vi "MFP3D Acquired Data.vi"() -> ()   [LabVIEW 2016]
uses:
  <userlib>/LevyLab/Relay Box/Type_defs/Resistor--enum.ctl
  <vilib>/DAQmx/read.llb/DAQmx Read (Analog 1D DBL NChan 1Samp).vi
  subVIs/Driver Variables_MFP3D.vi
  <vilib>/DAQmx/create/channels.llb/DAQmx Create Channel (AI-Voltage-Basic).vi
  <vilib>/DAQmx/configure/timing.llb/DAQmx Timing (Sample Clock).vi
  <vilib>/DAQmx/miscellaneous.llb/DAQmx Fill In Error Info.vi
  <vilib>/Platform/TimedLoop/XDataNode/XDataNode.xnode
  <vilib>/Platform/TimedLoop/XDataNode/timing_clust.ctl
  <vilib>/Platform/TimedLoop/XDataNode/nitl_modes.ctl
  <vilib>/Platform/TimedLoop/XDataNode/wakeup.ctl
  <vilib>/Platform/TimedLoop/XDataNode/XDNodeRunTimeDep.lvlib
panel:
  in  "Reset Graphs":bool
  in  "Data Queue":refnum<queue>
  in  "Skip Back Button":bool
  in  "FF Speed":dbl=2.0
  in  "Progress":dbl(slide)=0.002 scale=0.0..1435.0
  in  "Seek Forward Button":bool
  in  "Media Stop Button":bool
  in  "Play Button":bool
  in  "Tabs":T1(tab)
  in  "Lockin Information":T2={"SR7265 Sensitivity (A)"=5e-07, "Excitation Voltage (V)"=0.1, "SR810 Sensitivity (A)"=0.1, "Femto Gain (V/A)"=1.0, "Frequency (Hz)"=27.0}
  in  "Channel 1 (z, x, y, defl, Vtip, 4t I, 4t V)":tag="Dev1/ai0:5"
  in  "TDMS File Name":string="SA02821"
  in  "TDMS Output Folder":path=path "P:/users1/Yuhe/cypher tdms"
  out "TDMS Path Result":path
  in  "View Data After?":bool
  out "Z Value":cluster{"Y":dbl[], "Y":dbl[]}[](graph)
  out "X Position":cluster{"Y":dbl[], "Y":dbl[]}[](graph)
  out "Y Position":cluster{"Y":dbl[], "Y":dbl[]}[](graph)
  out "Tip Deflection":cluster{"Y":dbl[], "Y":dbl[]}[](graph)
  out "Tip Voltage":cluster{"Y":dbl[], "Y":dbl[]}[](graph)
  out "2-Terminal Conductance":cluster{"Y":dbl[], "Y":dbl[]}[](graph)
  out "2-Terminal Resistance":cluster{"Y":dbl[], "Y":dbl[]}[](graph)
  out "4-Terminal Conductance":cluster{"Y":dbl[], "Y":dbl[]}[](graph)
  out "4-Terminal Resistance":cluster{"Y":dbl[], "Y":dbl[]}[](graph)
  in  "Background Image":refnum<vi>
  in  "Inkscape File (.svg)":refnum<vi>
  in  "Run":refnum<vi>
  in  "Abort":refnum<vi>
  in  "Lithography Data":T4(array[cluster])
  # "FUTURE: will be used for TDMS playback"
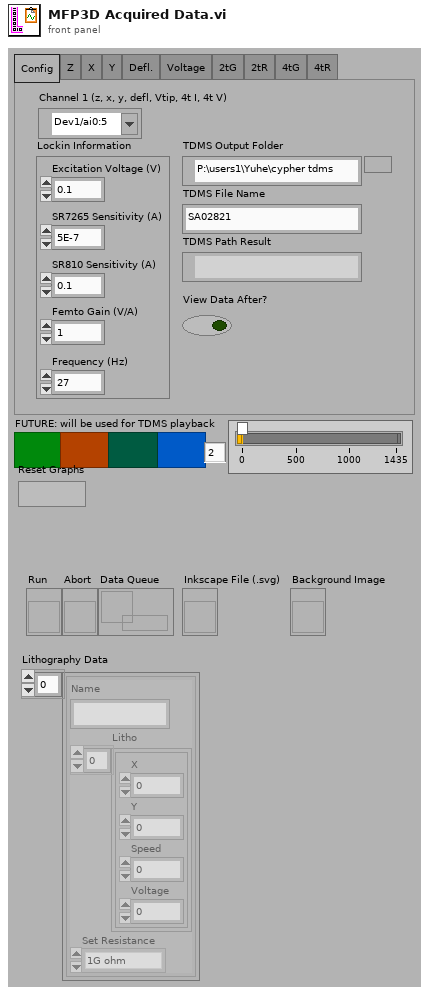
[diagram p1: front panel]
types:
  T1 = enum32{"Config", "Z", "X", "Y", "Defl.", "Voltage", "2tG", "2tR", "4tG", "4tR"}
  T2 = cluster{"SR7265 Sensitivity (A)":dbl, "Excitation Voltage (V)":dbl, "SR810 Sensitivity (A)":dbl, "Femto Gain (V/A)":dbl, "Frequency (Hz)":dbl}
  T3 = typedef "Resistor--enum.ctl" = enum16{"open", "discharge tip", "0 ohms", "100k ohm", "10M ohm", "1G ohm"}
  T4 = cluster{"Name":string, "Litho":cluster{"X":dbl, "Y":dbl, "Speed":dbl, "Voltage":dbl}[], "Set Resistance":T3}[]
  T5 = typedef "XDNodeRunTimeDep.lvlib/timing_clust.ctl" = cluster{"Expected End [f-1]":u64, "Actual End [f-1]":u64, "Finished Late? [f-1]":bool, "Expected End [i-1]":u64, "Actual End [i-1]":u64, "Finished Late? [i-1]":bool, "Expected Start [i]":u64, "Actual Start [i]":u64, "Expected Start [f]":u64, "Actual Start [f]":u64, "Source Name":string, "Structure Name":string, "Period":i64, "Deadline":i64, "Offset":i64, "Start":i64, "Priority":i32, "Timeout":i32, "Mode":T6, "Wakeup Reason":T7, "Error":errorcluster, "Source Type":string, "Secondary Source Type":string, "Global End Time":u64, "Global Start Time":u64, "Frame Duration":u64, "Iteration Duration":u64, "Assigned CPU":i32, "I/O Scan Engine Mode":u32}
  T6 = typedef "XDNodeRunTimeDep.lvlib/nitl_modes.ctl" = enum32{"No Change", "Process missed periods, maintain original phase", "Discard missed periods, maintain original phase", "Process missed periods, ignore original phase", "Discard missed periods, ignore original phase"}
  T7 = typedef "XDNodeRunTimeDep.lvlib/wakeup.ctl" = enum32{"Normal", "Aborted", "Asynchronous wakeup", "Timing source error", "Timed loop error", "Timeout"}
  T8 = cluster{"Result":dbl, "Result":dbl, "Result":dbl, "Result":dbl, "Result":dbl, "Result":dbl}
  T9 = cluster{"SR7265 Sensitivity (A)":dbl, "Excitation Voltage (V)":dbl, "Femto Gain (V/A)":dbl, "SR810 Sensitivity (A)":dbl}
  T10 = cluster{"x":dbl, "y":dbl, "Voltage":dbl, "Voltage":dbl}
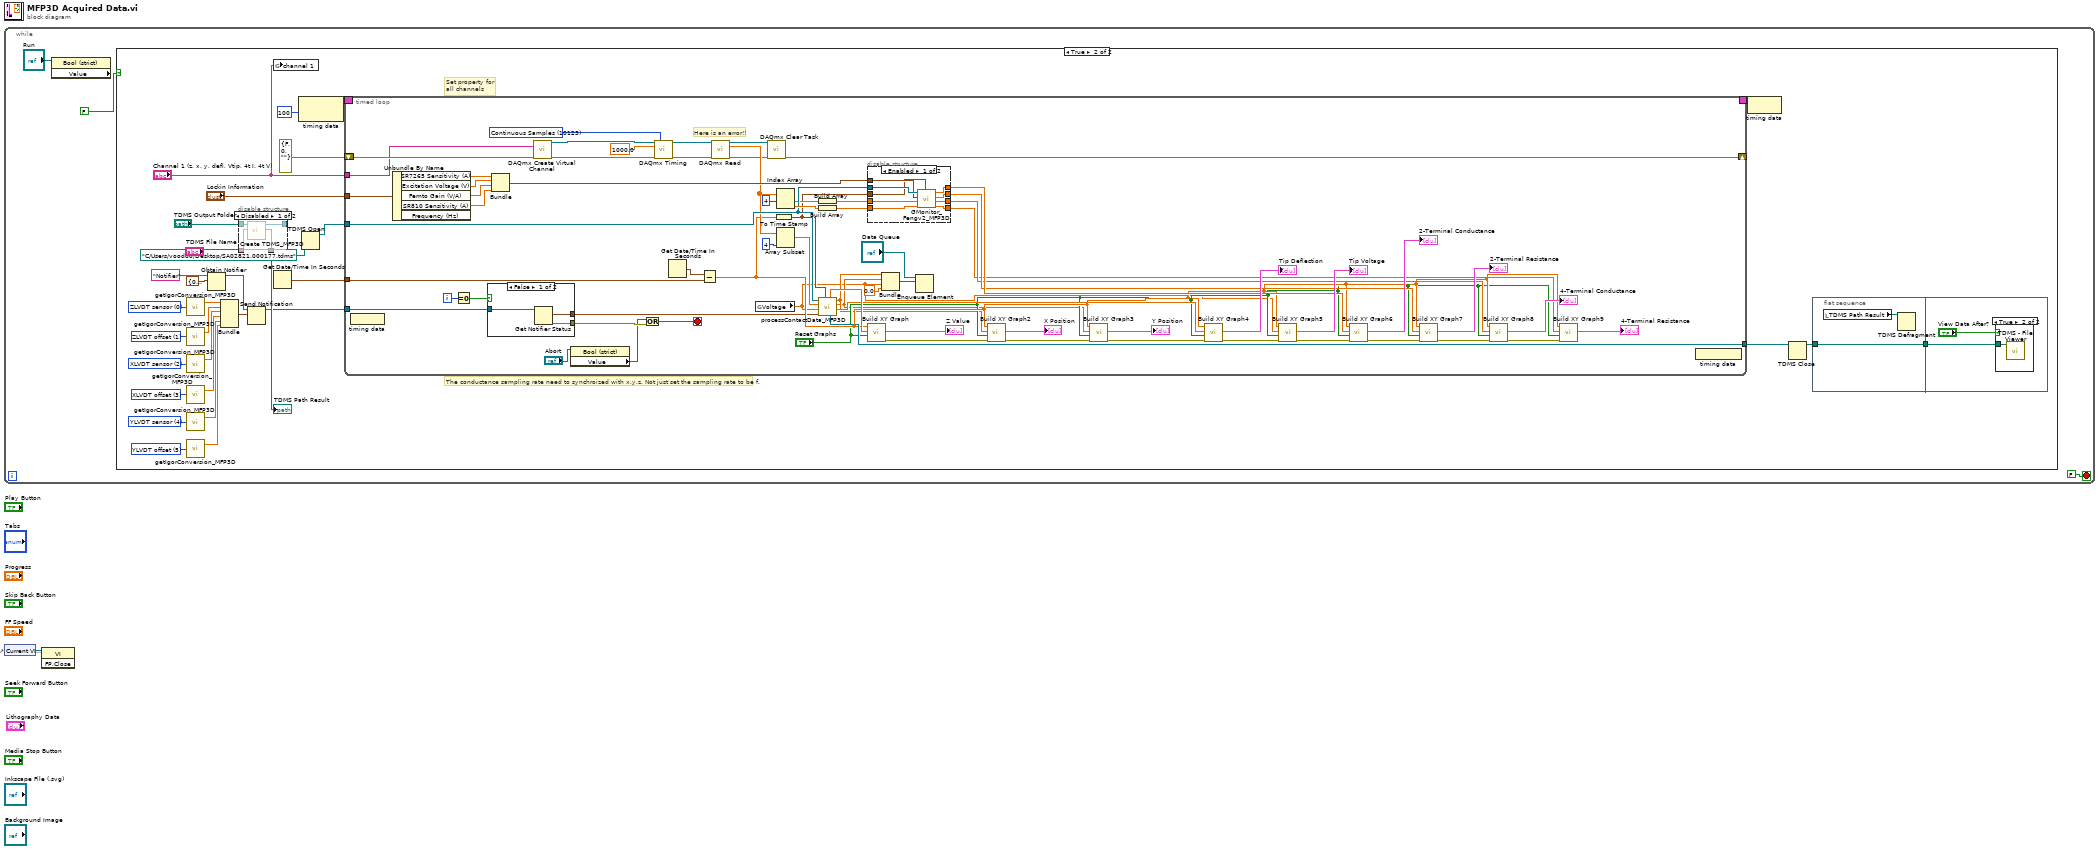
[diagram p0: block diagram]
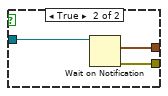
[diagram p6: hidden frame]
diagram:
  n1 = while {
    stop <- FALSE stop-if-true
    n2 = property class="Bool (strict)" props=["Value"](reference="Run") -> ()  [unwired: 1 in, 3 out]
    n3 = case shown="True" FALSE {
      frame False {
      }
      frame True {
        w18 = 5 items=["ZLVDT sensor", "ZLVDT offset", "XLVDT sensor", "XLVDT offset", "YLVDT sensor", "YLVDT offset", "DEFL"] ("index")
        w19 = 4 items=["ZLVDT sensor", "ZLVDT offset", "XLVDT sensor", "XLVDT offset", "YLVDT sensor", "YLVDT offset", "DEFL"] ("index")
        w20 = 3 items=["ZLVDT sensor", "ZLVDT offset", "XLVDT sensor", "XLVDT offset", "YLVDT sensor", "YLVDT offset", "DEFL"] ("index")
        w21 = 2 items=["ZLVDT sensor", "ZLVDT offset", "XLVDT sensor", "XLVDT offset", "YLVDT sensor", "YLVDT offset", "DEFL"] ("index")
        w22 = 1 items=["ZLVDT sensor", "ZLVDT offset", "XLVDT sensor", "XLVDT offset", "YLVDT sensor", "YLVDT offset", "DEFL"] ("index")
        w23 = 0 items=["ZLVDT sensor", "ZLVDT offset", "XLVDT sensor", "XLVDT offset", "YLVDT sensor", "YLVDT offset", "DEFL"] ("index")
        # "Set property for \nall channels"
        # "The conductance sampling rate need to synchroized with x,y,z. Not just set the sampling rate to be f."
        n4 = call "getIgorConversion_MFP3D.vi"("index"=w23) -> ("Result"=w17:dbl)  [unwired: 1 out]
        n5 = call "getIgorConversion_MFP3D.vi"("index"=w22) -> ("Result"=w16:dbl)  [unwired: 1 out]
        n6 = call "getIgorConversion_MFP3D.vi"("index"=w21) -> ("Result"=w15:dbl)  [unwired: 1 out]
        n7 = call "getIgorConversion_MFP3D.vi"("index"=w20) -> ("Result"=w14:dbl)  [unwired: 1 out]
        n8 = call "getIgorConversion_MFP3D.vi"("index"=w19) -> ("Result"=w13:dbl)  [unwired: 1 out]
        n9 = call "getIgorConversion_MFP3D.vi"("index"=w18) -> ("Result"=w12:dbl)  [unwired: 1 out]
        n10 = Obtain Notifier(name (unnamed)="Notifier", notification data type=cluster{dbl, dbl, dbl, dbl, dbl, dbl} {0.0, 0.0, 0.0, 0.0, 0.0, 0.0}) -> (notifier out=w10:refnum<notifier>)  [unwired: 2 in, 2 out]
        n11 = Bundle("Result"=w17, "Result"=w16, "Result"=w15, "Result"=w14, "Result"=w13, "Result"=w12) -> (w11:T8)  [unwired: 1 in]
        n12 = disable-structure shown="Disabled" {
          disable-tunnel: "TDMS Output Folder" -> [w40 _]
          disable-tunnel: "TDMS File Name" -> [w39 _]
          disable-tunnel: [w38 _] -> w31
          disable-tunnel: [w37 _] -> _
          frame Disabled {
            n13 = call <vilib>:"Create TDMS_MFP3D.vi"("TDMS File Name"=w39, "TDMS Output Folder"=w40) -> ("modified path"=w38:path, "Refnum out"=w37:refnum<k34>)  [unwired: 8 in]
          }
          frame Enabled {
          }
        }
        "TDMS Path Result" <- w31
        n14 = Send Notification(notification=w11, notifier=w10) -> (notifier out=w8:refnum<notifier>)  [unwired: 1 in, 1 out]
        n15 = global write "Driver Variables_MFP3D.vi" "channel 1"("Channel 1 (z, x, y, defl, Vtip, 4t I, 4t V)") -> ()
        n16 = Get Date/Time In Seconds() -> (seconds since 1Jan1904=w27:timestamp)
        n17 = node-c288(100) -> (w36:T5)
        n18 = TDMS Open(11:path "C:/Users/voodoo/Desktop/SA02821.000177.tdms" ("file path")) -> (3:w6:refnum<k34>)  [unwired: 6 in, 1 out]
        n19 = timed-loop {
          timing: w36 -> [_]
          timing-out: [_] -> w35
          tunnel: w8 -> [w112]
          tunnel: w6 -> [w107]
          shift-right: [w69] -> _
          shift-left: errorcluster {"status"=FALSE, "code"=0, "source"=""} ("error out") -> [w63]
          tunnel: "Lockin Information" -> [w106]
          tunnel: [w108] -> w29
          tunnel: w27 -> [w100]
          tunnel: "Channel 1 (z, x, y, defl, Vtip, 4t I, 4t V)" -> [w60]
          i -> [w114]
          stop <- w53 stop-if-true
          w67 = 10123 items=["Finite Samples"=10178, "Continuous Samples"=10123, "Hardware Timed Single Point"=12522] ("sample mode")
          # "Here is an error!!"
          n20 = node-c288() -> ()  [unwired: 1 in]
          n21 = Unbundle By Name(w106) -> ("SR7265 Sensitivity (A)"=w101:dbl, "Excitation Voltage (V)"=w105:dbl, "Femto Gain (V/A)"=w104:dbl, "SR810 Sensitivity (A)"=w103:dbl)  [unwired: 1 out]
          n22 = Equal To 0?(x=w114) -> (x = 0?=w113:bool)
          n23 = case shown="False" w113 {
            tunnel: w112 -> [w126 w129]
            tunnel: [w125 w128] -> w55
            tunnel: [w124 w127] -> w57
            frame False {
              n24 = Get Notifier Status(notifier=w126) -> (current notification=w124:cluster{dbl, dbl, dbl, dbl, dbl, dbl}, error out=w125:errorcluster)  [unwired: 1 in, 3 out]
            }
            frame True {
              n25 = Wait on Notification(notifier=w129) -> (notification=w127:cluster{dbl, dbl, dbl, dbl, dbl, dbl}, error out=w128:errorcluster)  [unwired: 3 in, 2 out]
            }
          }
          n26 = Bundle("SR7265 Sensitivity (A)"=w101, "Excitation Voltage (V)"=w105, "Femto Gain (V/A)"=w104, "SR810 Sensitivity (A)"=w103) -> (w102:T9)  [unwired: 1 in]
          n27 = call-poly <vilib>:"DAQmx Create Virtual Channel.vi"("physical channels"=w60, "error in"=w63) -> ("task out"=w66:refnum<k21>, "error out"=w65:errorcluster)  [unwired: 12 in]
          n28 = property class="Bool (strict)"(reference="Abort") -> ("Value"=w54:bool)  [unwired: 1 in, 2 out]
          n29 = Or(x=w54, y=w55) -> (x .or. y?=w53:bool)
          n30 = call-poly <vilib>:"DAQmx Timing.vi"("task/channels in"=w66, "sample mode"=w67, "rate"=1000.0, "error in"=w65) -> ("task out"=w64:refnum<k21>, "error out"=w62:errorcluster)  [unwired: 10 in]
          n31 = Get Date/Time In Seconds() -> (seconds since 1Jan1904=w97:timestamp)
          n32 = Subtract(x=w97, y=w100) -> (x-y=w59:dbl)
          n33 = call-poly <vilib>:"DAQmx Read.vi"("task/channels in"=w64, "error in"=w62) -> ("task out"=w61:refnum<k21>, "data"=w71:dbl[], "error out"=w70:errorcluster)  [unwired: 11 in]
          n34 = global read "Driver Variables_MFP3D.vi" "Voltage"() -> (w49:dbl)
          n35 = call <vilib>:"DAQmx Clear Task.vi"("task in"=w61, "error in"=w70) -> ("error out"=w69:errorcluster)  [unwired: 13 in]
          n36 = To Time Stamp(1:w59) -> (0:w58:timestamp)
          n37 = Index Array(array=w71, index #1=4) -> (element #1=w83:dbl, element #2=w110:dbl)  [unwired: 1 in]
          n38 = Array Subset(array=w71, length=4) -> (w72:dbl[])  [unwired: 1 in]
          n39 = Build Array(w83) -> (w82:dbl[])
          n40 = Build Array(w110) -> (w109:dbl[])
          n41 = call "processContactData_MFP3D.vi"("tdms file"=w107, "data"=w72, "tip voltage"=w49, "lvdt"=w57, "time stamp"=w58) -> ("z"=w98:dbl, "tdms file out"=w108:refnum<k34>, "x"=w51:dbl, "y"=w50:dbl, "deflection"=w93:dbl)  [unwired: 1 out]
          n42 = disable-structure shown="Enabled" {
            disable-tunnel: w109 -> [w123 _]
            disable-tunnel: w107 -> [w122 _]
            disable-tunnel: w102 -> [w121 _]
            disable-tunnel: w58 -> [w120 _]
            disable-tunnel: [w119 _] -> w90
            disable-tunnel: [w118 _] -> w88
            disable-tunnel: [w117 _] -> w85
            disable-tunnel: [w116 _] -> w84
            disable-tunnel: w82 -> [w115 _]
            frame Enabled {
              n43 = call "GMonitor_Fengv2_MFP3D.vi"("Time Stamp"=w120, "v1"=w123, "v0"=w115, "lockin information"=w121, "tdms file"=w122) -> ("FtR"=w116:dbl, "FtG"=w117:dbl, "TtR"=w118:dbl, "TtG"=w119:dbl)  [unwired: 1 out]
            }
            frame Disabled {
            }
          }
          n44 = call "Build XY Graph"("Reset"="Reset Graphs", "Y Input"=w98, "X Input"=w59) -> ("error out"=w81:errorcluster, "XY Graph"=→"Z Value":cluster{"X":dbl[], "Y":dbl[]}[])  [unwired: 7 in]
          n45 = Bundle("x"=w51, "y"=w50, "Voltage"=w49, "Voltage"=0.0) -> (w47:T10)  [unwired: 1 in]
          n46 = Enqueue Element(queue="Data Queue", element=w47) -> ()  [unwired: 2 in, 3 out]
          n47 = call "Build XY Graph2"("error in (no error)"=w81, "Reset"="Reset Graphs", "Y Input"=w51, "X Input"=w59) -> ("error out"=w80:errorcluster, "XY Graph"=→"X Position":cluster{"X":dbl[], "Y":dbl[]}[])  [unwired: 6 in]
          n48 = call "Build XY Graph3"("error in (no error)"=w80, "Reset"="Reset Graphs", "Y Input"=w50, "X Input"=w59) -> ("error out"=w79:errorcluster, "XY Graph"=→"Y Position":cluster{"X":dbl[], "Y":dbl[]}[])  [unwired: 6 in]
          n49 = call "Build XY Graph4"("error in (no error)"=w79, "Reset"="Reset Graphs", "Y Input"=w93, "X Input"=w59) -> ("error out"=w78:errorcluster, "XY Graph"=→"Tip Deflection":cluster{"X":dbl[], "Y":dbl[]}[])  [unwired: 6 in]
          n50 = call "Build XY Graph5"("error in (no error)"=w78, "Reset"="Reset Graphs", "Y Input"=w49, "X Input"=w59) -> ("error out"=w77:errorcluster, "XY Graph"=→"Tip Voltage":cluster{"X":dbl[], "Y":dbl[]}[])  [unwired: 6 in]
          n51 = call "Build XY Graph6"("error in (no error)"=w77, "Reset"="Reset Graphs", "Y Input"=w90, "X Input"=w59) -> ("error out"=w76:errorcluster, "XY Graph"=→"2-Terminal Conductance":cluster{"X":dbl[], "Y":dbl[]}[])  [unwired: 6 in]
          n52 = call "Build XY Graph7"("error in (no error)"=w76, "Reset"="Reset Graphs", "Y Input"=w88, "X Input"=w59) -> ("error out"=w75:errorcluster, "XY Graph"=→"2-Terminal Resistance":cluster{"X":dbl[], "Y":dbl[]}[])  [unwired: 6 in]
          n53 = call "Build XY Graph8"("error in (no error)"=w75, "Reset"="Reset Graphs", "Y Input"=w85, "X Input"=w59) -> ("error out"=w74:errorcluster, "XY Graph"=→"4-Terminal Conductance":cluster{"X":dbl[], "Y":dbl[]}[])  [unwired: 6 in]
          n54 = call "Build XY Graph9"("error in (no error)"=w74, "Reset"="Reset Graphs", "Y Input"=w84, "X Input"=w59) -> ("XY Graph"=→"4-Terminal Resistance":cluster{"X":dbl[], "Y":dbl[]}[])  [unwired: 6 in, 1 out]
          n55 = node-c288() -> ()  [unwired: 1 out]
        }
        n56 = node-c288(w35) -> ()
        n57 = TDMS Close(11:w29) -> (3:w28:path)  [unwired: 1 in, 1 out]
        n58 = flat-sequence {
          tunnel: w28 -> [w42]
          tunnel: [w42] -> w34
          tunnel: w34 -> [w44]
          frame #0 {
            n59 = local read "TDMS Path Result"() -> (w41:path)
            n60 = TDMS Defragment(7:w41) -> ()  [unwired: 1 in, 1 out]
          }
          frame #1 {
            n61 = case shown="True" "View Data After?" {
              tunnel: w44 -> [_ w45]
              frame False {
              }
              frame True {
                n62 = call <vilib>:"TDMS - File Viewer.vi"("file path"=w45) -> ()  [unwired: 5 in, 2 out]
              }
            }
          }
        }
      }
    }
  }
  n63 = control-ref of="Current VI Reference"() -> (w1:refnum<vi>)
  n64 = invoke class="VI" method="FP.Close"(reference=w1) -> ()  [unwired: 2 in, 3 out]
